vi "add_JointCommandMode.vi"(4 "Mode":enum16{"Position", "Velocity", "Effort"}(ring), 5 "msg in":string) -> (2 "msg out":string)   [LabVIEW 2010]
uses:
  <userlib>/ROSforLV_0.1/ROS/MessageBuilding/Primitives/subs/u8Scalar.vi
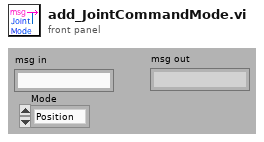
[diagram p1: front panel]
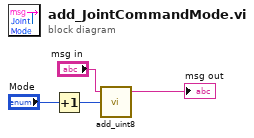
[diagram p0: block diagram]
diagram:
  n1 = Increment(x="Mode") -> (x+1=w3:enum16{"Position", "Velocity", "Effort"})
  n2 = call-poly <userlib>:"add_uint8.vi"("Numeric"=w3, "msg in"="msg in") -> ("msg out"=→"msg out":string)  [unwired: 3 in]
